vi "BP FilterCoeffs.vi"(1 "sample rate MHz":dbl, 4 "Filter Prams":T1={"low cutoff"=5.0, "order"=81, "high cutoff"=35.0}, 5 "filter type":T2(ring)=enum."Bandpass") -> (0 "FIR Windowed Coefficients":dbl[](array[numeric]))   [LabVIEW 2022 SP3]
uses:
  <vilib>/Analysis/4window.llb/windowTd.ctl
  <vilib>/Analysis/NI_AALBase.lvlib
  <vilib>/Analysis/NI_AALPro.lvlib
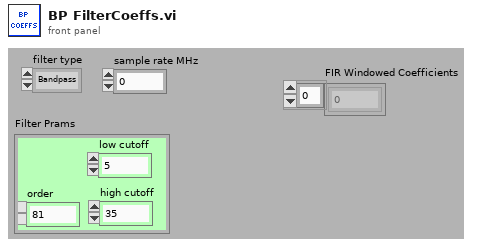
[diagram p1: front panel]
types:
  T1 = cluster{"low cutoff":dbl, "order":i32, "high cutoff":dbl}
  T2 = enum32{"Lowpass", "Highpass", "Bandpass", "Bandstop"}
  T3 = typedef "NI_AALPro.lvlib/windowTd.ctl" = u32
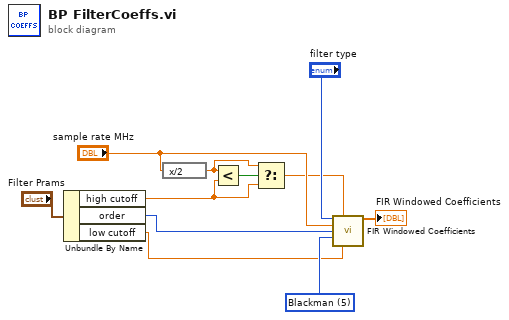
[diagram p0: block diagram]
diagram:
  w8 = T3 5 items=["Rectangle"=0, "Hanning"=1, "Hamming"=2, "Blackman-Harris"=3, "Exact Blackman"=4, "Blackman"=5, "Flat Top"=6, "4 Term B-Harris "=7, "7 Term B-Harris"=8, "Low Sidelobe"=9, "Blackman Nuttall"=11, "Triangle"=30, "Bartlett-Hanning"=31, "Bohman"=32, "Parzen"=33, "Welch"=34, "Kaiser"=60, "Dolph-Chebyshev"=61, "Gaussian"=62] ("window")
  n1 = Unbundle By Name("Filter Prams") -> ("high cutoff"=w3:dbl, "order"=w9:i32, "low cutoff"=w6:dbl)
  n2 = expression code="x/2"("sample rate MHz") -> (w4:dbl)
  n3 = Less?(x=w4, y=w3) -> (x < y?=w5:bool)
  n4 = Select(t=w4, s=w5, f=w3) -> (s? t:f=w1:dbl)
  n5 = call <vilib>:"FIR Windowed Coefficients.vi"("filter type"="filter type", "high cutoff freq: fh"=w1, "sampling freq: fs"="sample rate MHz", "taps"=w9, "window"=w8, "low cutoff freq: fl"=w6) -> ("FIR Windowed Coefficients"=→"FIR Windowed Coefficients":dbl[])  [unwired: 2 in, 7 out]
